vi "to string.vi"(8 "error in":errorcluster, 11 "channel in":refnum<class "TBM channel.lvclass">) -> (0 "error out":errorcluster, 1 "channel data":string, 2 "identifier":string, 3 "channel out":refnum<class "TBM channel.lvclass">)   [LabVIEW 2013, in "TBM channel.lvclass"]
uses:
  TBM channel.lvclass
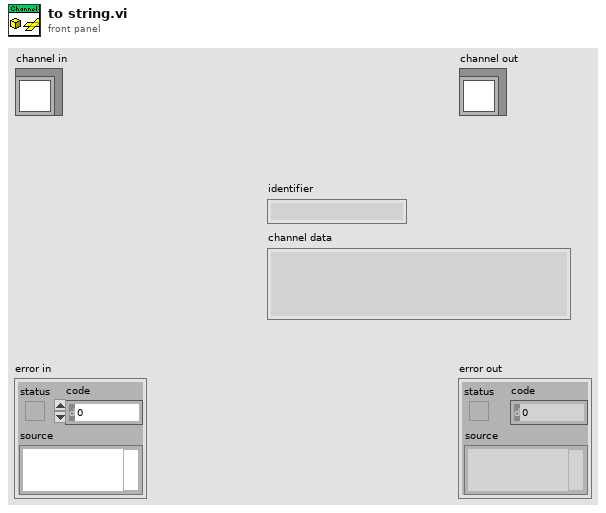
[diagram p1: front panel]
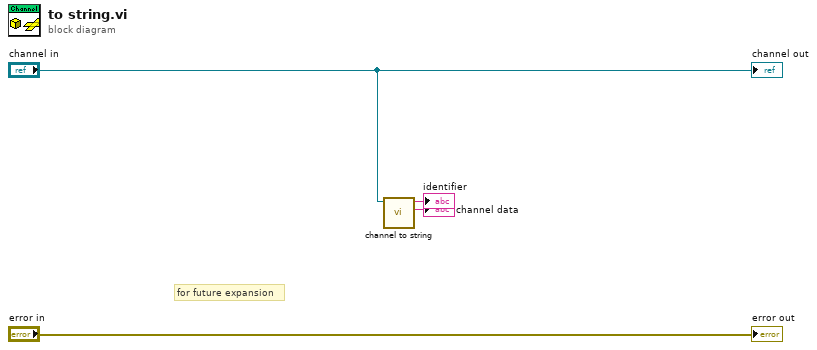
[diagram p0: block diagram]
diagram:
  # "for future expansion"
  n1 = call "channel to string.vi"("channel in"="channel in") -> ("channel data"=→"channel data":string, "identifier"=→"identifier":string)  [unwired: 9 in]
  "error out" <- "error in"
  "channel out" <- "channel in"
